vi "GetPropertyIndex.vi"(0 "JSON":string, 1 "compare string":string="NI.Scratchpad64.U64") -> (14 "Item offset":i32)   [LabVIEW 2018]
uses:
  54ead8a2-d1f8-4c70-ae5c-dbc70cd2a8d0.vi
  <vilib>/JDP Science/JSONtext/String Subset.vi
  <vilib>/JDP Science/JSONtext/support/Strip Quotes and Unescape.vi
  <vilib>/JDP Science/JSONtext/Parsing/Parse Full Path or Item Name.vi
  <vilib>/JDP Science/JSONtext/Offset/Find Item Locations by Path.vi
  <vilib>/JDP Science/JSONtext/support/Unescape JSON string.vi
  <vilib>/JDP Science/JSONtext/JSON text to Variant.vi
  <vilib>/JDP Science/JSONtext/JSONtext.lvlib
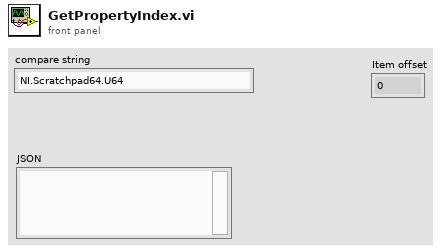
[diagram p1: front panel]
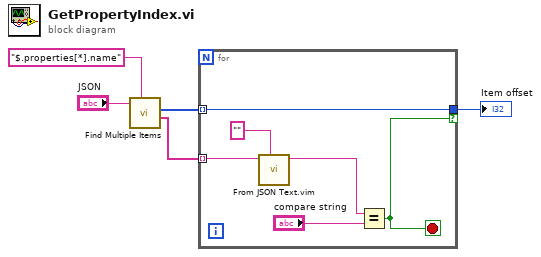
[diagram p0: block diagram]
diagram:
  n1 = call <vilib>:"Find Multiple Items.vi"("$Path or Item Name"="$.properties[*].name", "JSON"="JSON") -> ("<JSON>"=w2:string[], "Item Offsets"=w4:i32[])  [unwired: 6 in, 2 out]
  n2 = for {
    tunnel: w4 -> [w10] mode=indexing
    tunnel: [w10] -> w3 if=w9
    tunnel: w2 -> [w8] mode=indexing
    stop <- w9 stop-if-true
    n3 = call "From JSON Text.vim"("Data Type and Default Value"="", "JSON"=w8) -> ("Data out"=w6:string)  [unwired: 8 in, 1 out]
    n4 = Equal?(x=w6, y="compare string") -> (x = y?=w9:bool)
  }
  "Item offset" <- w3
